vi "Type Cast.vi"(1 "Module in":T1) -> (0 "Module":T2)   [LabVIEW 2022 SP3, in "Core.lvlib" / "Module.lvlib"]
uses:
  Module.lvlib
  Controls/Module.ctl
  Controls/Instance.ctl
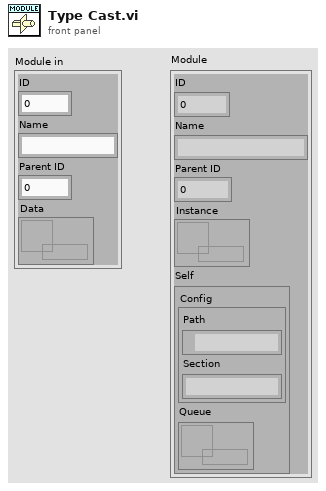
[diagram p1: front panel]
types:
  T1 = cluster{"ID":i32, "Name":string, "Parent ID":i32, "Data":refnum<data-value>}
  T2 = typedef "Core.lvlib/Module.lvlib/Module.ctl" = cluster{"ID":i32, "Name":string, "Parent ID":i32, "Instance":refnum<data-value>, "Self":T3}
  T3 = typedef "Core.lvlib/Module.lvlib/Instance.ctl" = cluster{"Config":cluster{"Path":path, "Section":string}, "Queue":refnum<queue>}
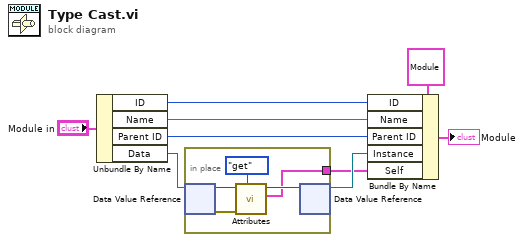
[diagram p0: block diagram]
diagram:
  n1 = Unbundle By Name("Module in") -> ("ID"=w6:i32, "Name"=w5:string, "Parent ID"=w4:i32, "Data"=w3:refnum<data-value>)
  n2 = in-place {
    in-place-border: [w11] -> w1
    n3 = in-place-dvr #1(w3) -> (w14:variant, w13:errorcluster)
    n4 = call "Attributes.vi"("Action"=enum8{"get", "set"}."get", "error in (no error)"=w13, "Instance in"=w14) -> ("Self out"=w11:T3, "Instance out"=w12:variant)  [unwired: 6 in, 1 out]
    n5 = in-place-dvr #1(w12) -> (w2:refnum<data-value>)  [unwired: 1 out]
  }
  n6 = Bundle By Name(cluster=T2 {"ID"=0, "Name"="", "Parent ID"=0, "Instance"=refnum, "Self"={"Config"={"Path"=path "", "Section"=""}, "Queue"=refnum}} ("Module"), "ID"=w6, "Name"=w5, "Parent ID"=w4, "Instance"=w2, "Self"=w1) -> (→"Module":T2)
